vi "ALTS-2015 Create Default User Info.vi"(8 "error in":errorcluster) -> (0 "error out":errorcluster)   [LabVIEW 2013]
uses:
  <vilib>/Utility/config.llb/NI_LVConfig.lvlib
  Controls/ALTS-2015 User Group Enum2.ctl
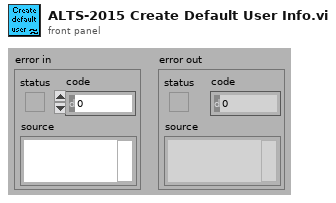
[diagram p1: front panel]
types:
  T1 = typedef "ALTS-2015 User Group Enum2.ctl" = enum16{"Administrator", "Super User", "Operator"}
  T2 = typedef "NI_LVConfig.lvlib/Config Data RefNum.ctl" = refnum<k1>
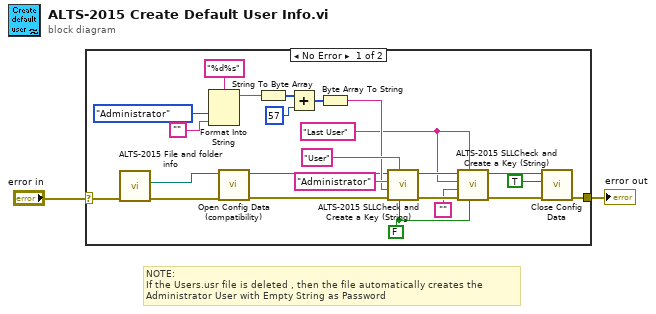
[diagram p0: block diagram]
diagram:
  # "NOTE:\nIf the Users.usr file is deleted , then the file automatically creates the Administrator User with Empty String as Password"
  n1 = case shown="No Error" "error in" {
    selector: "error in" -> [w5 w27]
    tunnel: [w10 w27] -> w1
    frame No Error {
      w17 = "Last User"
      w24 = FALSE ("write raw string? (F)")
      n2 = call "ALTS-2015 File and folder info.vi"("error in (no error)"=w5) -> ("error out"=w6:errorcluster, "INI file path"=w3:path)  [unwired: 5 in, 4 out]
      n3 = Format Into String(format string="%d%s", ALTS-2015_User_Group_Enum2."Administrator" ("User Group"), "") -> (resulting string=w4:string)  [unwired: 2 in, 1 out]
      n4 = call <vilib>:"Open Config Data (compatibility).vi"("error in (no error)"=w6, "configuration file path"=w3) -> ("error out"=w14:errorcluster, "refnum"=w15:T2)  [unwired: 7 in, 1 out]
      n5 = String To Byte Array(string=w4) -> (unsigned byte array=w23:u8[])
      n6 = Add(x=w23, y=57) -> (x+y=w21:i32[])
      n7 = Byte Array To String(unsigned byte array=w21) -> (string=w20:string)
      n8 = call "ALTS-2015 SLLCheck and Create a Key (String).vi"("Update Value? (F)"=w24, "Section"="User", "error in (no error)"=w14, "Default Value"=w20, "Key"="Administrator", "File Refnum in"=w15) -> ("error out"=w19:errorcluster, "File Refnum out"=w18:T2)  [unwired: 4 in]
      n9 = call "ALTS-2015 SLLCheck and Create a Key (String).vi"("Update Value? (F)"=w24, "Section"=w17, "error in (no error)"=w19, "Default Value"="", "Key"=w17, "File Refnum in"=w18) -> ("error out"=w13:errorcluster, "File Refnum out"=w12:T2)  [unwired: 4 in]
      n10 = call <vilib>:"Close Config Data.vi"("error in (no error)"=w13, "write file if changed (T)"=TRUE ("write configuration file? (F)"), "refnum"=w12) -> ("error out"=w10:errorcluster)  [unwired: 7 in, 1 out]
    }
    frame Error {
    }
  }
  "error out" <- w1
